vi "Ball Intake Piston.vi"() -> ()   [LabVIEW 2019]
uses:
  <vilib>/Rock Robotics/WPI/Solenoid/WPI_SolenoidValue.ctl
  <vilib>/Rock Robotics/WPI/Solenoid/Deprecated/WPI_SolenoidGetBool.vi
  <vilib>/Rock Robotics/WPI/Solenoid/WPI_SolenoidSetEnum.vi
panel:
  in  "Ball Intake Piston":bool
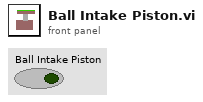
[diagram p1: front panel]
types:
  T1 = typedef "WPI_SolenoidValue.ctl" = enum16{"Off", "On", "Forward", "Reverse"}
  T2 = typedef "WPI_SolenoidDevRef.ctl" = cluster{"DevStatus":errorcluster, "Pneumatics Control Module":u8, "Forward Solenoid Channel":T3, "Reverse Solenoid Channel":T3}
  T3 = typedef "WPI_SolenoidChannel.ctl" = enum8{"Solenoid 0", "Solenoid 1", "Solenoid 2", "Solenoid 3", "Solenoid 4", "Solenoid 5", "Solenoid 6", "Solenoid 7", "Invalid"}
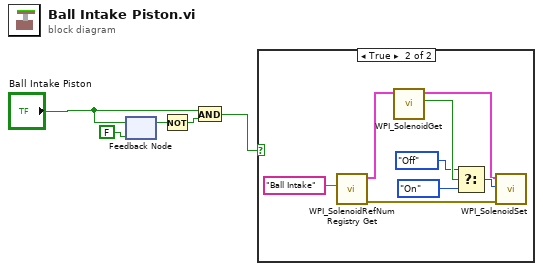
[diagram p0: block diagram]
diagram:
  n1 = feedback #1(FALSE ("Extend and Retract Arm")) -> (w4:bool)
  n2 = feedback-in #1("Ball Intake Piston") -> ()
  n3 = Not(x=w4) -> (.not. x?=w3:bool)
  n4 = And(x="Ball Intake Piston", y=w3) -> (x .and. y?=w1:bool)
  n5 = case shown="True" w1 {
    frame False {
    }
    frame True {
      n6 = call <vilib>:"WPI_SolenoidRefNum Registry Get.vi"("refnum name"="Ball Intake") -> ("error out"=w12:errorcluster, "SolenoidDevRef"=w10:T2)  [unwired: 9 in]
      n7 = call-poly <vilib>:"WPI_SolenoidGet.vi"("SolenoidDevRef"=w10) -> ("Value"=w13:bool, "SolenoidDevRef"=w9:T2)  [unwired: 8 in, 1 out]
      n8 = Select(t=WPI_SolenoidValue."Off", s=w13, f=WPI_SolenoidValue."On" ("Value")) -> (s? t:f=w11:T1)
      n9 = call-poly <vilib>:"WPI_SolenoidSet.vi"("error in (no error)"=w12, "Value"=w11, "SolenoidDevRef"=w9) -> ()  [unwired: 7 in, 2 out]
    }
  }
